vi "LVOOP is Same or Descendant Class Inline.vi"(1 "Possible Descendant Object":refnum<class>, 2 "Object":refnum<class>) -> (0 "Is Same Class or Descendant?":bool)   [LabVIEW 2019, in "BlueSerialization.lvlib" / "BlueSerializer.lvclass"]
uses:
  BlueSerializer.lvclass
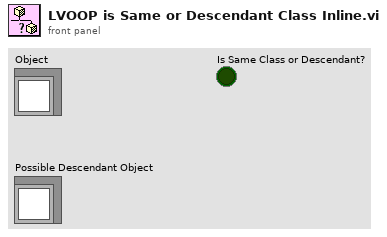
[diagram p1: front panel]
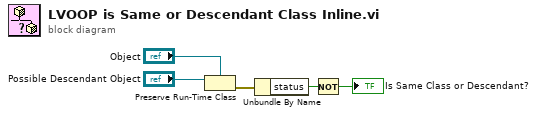
[diagram p0: block diagram]
diagram:
  n1 = Preserve Run-Time Class(object in="Possible Descendant Object", 2:"Object") -> (error out=w3:errorcluster)  [unwired: 1 in, 1 out]
  n2 = Unbundle By Name(w3) -> ("status"=w4:bool)
  n3 = Not(x=w4) -> (.not. x?=→"Is Same Class or Descendant?":bool)
